vi "ShowPeriodByTripTime.vi"(2 "Load":i32, 3 "Preload":i32, 4 "Trip":i32) -> (0 "Period":string, 1 "PeriodTime":i32)   [LabVIEW 2015]
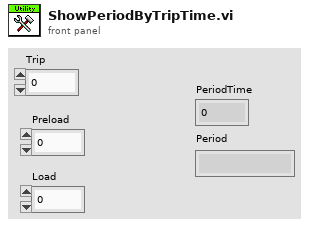
[diagram p1: front panel]
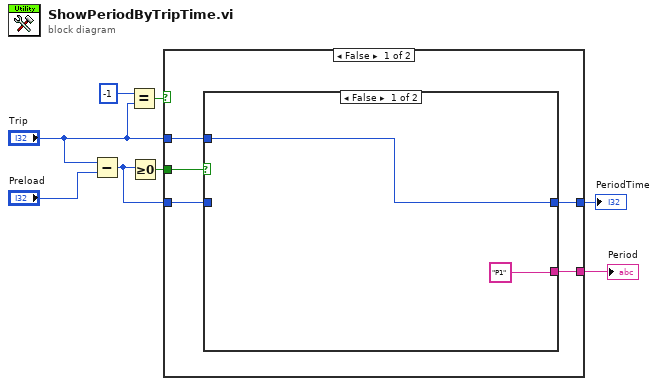
[diagram p0: block diagram]
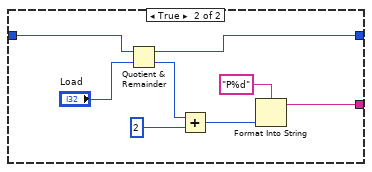
[diagram p2: hidden frame]
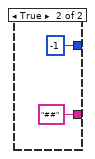
[diagram p3: hidden frame]
diagram:
  n1 = Subtract(x="Trip", y="Preload") -> (x-y=w6:i32)
  n2 = Equal?(x=-1, y="Trip") -> (x = y?=w1:bool)
  n3 = Greater Or Equal To 0?(x=w6) -> (x >= 0?=w7:bool)
  n4 = case shown="False" w1 {
    tunnel: w7 -> [w13 _]
    tunnel: w6 -> [w12 _]
    tunnel: [w11 -1 ("Trip")] -> w5
    tunnel: [w10 "##" ("Period")] -> w4
    tunnel: "Trip" -> [w9 _]
    frame False {
      n5 = case shown="False" w13 {
        tunnel: w12 -> [_ w23]
        tunnel: [w14 w21] -> w11
        tunnel: ["P1" ("Period") w16] -> w10
        tunnel: w9 -> [w14 _]
        frame False {
        }
        frame True {
          n6 = Quotient & Remainder(x=w23, y="Load") -> (x-y*floor(x/y)=w21:i32, floor(x/y)=w20:i32)
          n7 = Add(x=w20, y=2) -> (x+y=w17:i32)
          n8 = Format Into String(format string="P%d", w17) -> (resulting string=w16:string)  [unwired: 2 in, 1 out]
        }
      }
    }
    frame True {
    }
  }
  "Period" <- w4
  "PeriodTime" <- w5
